vi "Demo_Grab2.vi"() -> ()   [LabVIEW 2024]
doc: "Concurrently grab 2 video sources supported by QuickTime (internal, USB, FW, etc).\nSet Dialogs to 1 in Frame grabber settings to use the standard QT dialog.\n\nChris Salzmann © 1994-2003"
uses:
  <userlib>/ImageProcessing/QTLIB_2595_LV86/QT_Private.ctl
  <userlib>/ImageProcessing/QTLIB_2595_LV86/QT_Video.ctl
  <userlib>/ImageProcessing/QTLIB_2595_LV86/QT_FrameGrabber.ctl
panel:
  in  "Case Constant\n(See Context Help)":bool=TRUE
  in  "Hue 2":dbl(slide)=44.642857142857146 scale=0.0..100.0
  in  "Sat 2":dbl(slide)=39.285714285714285 scale=0.0..100.0
  in  "Bright 2":dbl(slide)=53.06122448979592 scale=0.0..100.0
  in  "Contr 2":dbl(slide)=57.142857142857146 scale=0.0..100.0
  in  "Sharp 2":dbl(slide) scale=0.0..100.0
  in  "Black l. 2":dbl(slide)=10.714285714285715 scale=0.0..100.0
  in  "White l. 2":dbl(slide)=80.61224489795919 scale=0.0..100.0
  out "QT Version 2":string="QuickTime v. 630 "
  out "CIN info 2":string="© Chris 94-2002, QT Fat-CIN, rev: 2576, FATQTCin.c, Jul 11 2003, 11:29:33"
  out "Picture 2":picture
  in  "Frame Grabber Settings 2":T1={"Name"="", "Digitizer"=2, "Input"=1, "Width"=320, "Height"=240, "Input format"=enum."NTSC", "Frame rate"=0.0, "Reserved"=0, "Dialogs"=0} {"Frame rate" format="%#1_6g"; "Dialogs" format="%.0b"}
  out "error out":errorcluster
  in  "White l.":dbl(slide)=80.61224489795919 scale=0.0..100.0
  in  "Black l.":dbl(slide)=51.78571428571429 scale=0.0..100.0
  in  "Sharp":dbl(slide)=12.5 scale=0.0..100.0
  in  "Contr":dbl(slide)=57.142857142857146 scale=0.0..100.0
  in  "Bright":dbl(slide)=53.06122448979592 scale=0.0..100.0
  in  "Sat":dbl(slide)=51.02040816326531 scale=0.0..100.0
  in  "Hue":dbl(slide)=50.0 scale=0.0..100.0
  out "Picture":picture
  in  "stop":bool
  in  "Frame Grabber Settings":T1={"Name"="", "Digitizer"=2, "Input"=0, "Width"=320, "Height"=240, "Input format"=enum."PAL", "Frame rate"=0.0, "Reserved"=0, "Dialogs"=0} {"Frame rate" format="%#1_6g"; "Dialogs" format="%.0b"}
  # "Concurrently grab 2 video sources supported by QuickTime(internal, USB, FW, etc)..\nSet Dialogs to 1 in Frame grabber settings to use the standard QT dialog.\n\nChris Salzmann © 1994-2005"
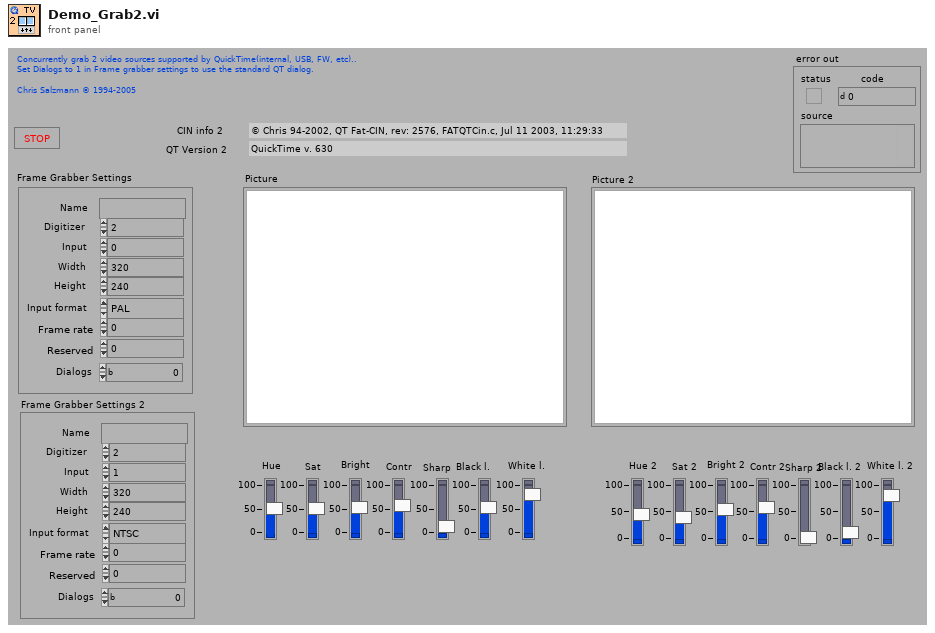
[diagram p1: front panel]
types:
  T1 = typedef "QT_FrameGrabber.ctl" = cluster{"Name":string, "Digitizer":i32, "Input":i32, "Width":i32, "Height":i32, "Input format":enum32{"NTSC", "PAL", "Secam"}, "Frame rate":dbl, "Reserved":i32, "Dialogs":u32}
  T2 = typedef "QT_Video.ctl" = cluster{"Color format":u32, "Hue":dbl, "Saturation":dbl, "Brightness":dbl, "Contrast":dbl, "Sharpness":dbl, "Black Level":dbl, "White Level":dbl, "Options":i32, "Dialogs":u32}
  T3 = typedef "QT_Private.ctl" = cluster{"reserved 1":i32, "reserved 2":i32, "reserved 3":i32, "reserved 4":i32}
  T4 = typedef "QT_Ref.ctl" = refnum<k1>
  T5 = typedef "QT_Image.ctl" = cluster{"Width":i32, "Height":i32, "Depth":i32, "data":u8[], "Compressed data":u8[], "Color table":u32[], "Duration":i32, "Options":i32, "Timestamp":i32, "ID":i32, "Reserved":i32, "Dialogs":u32}
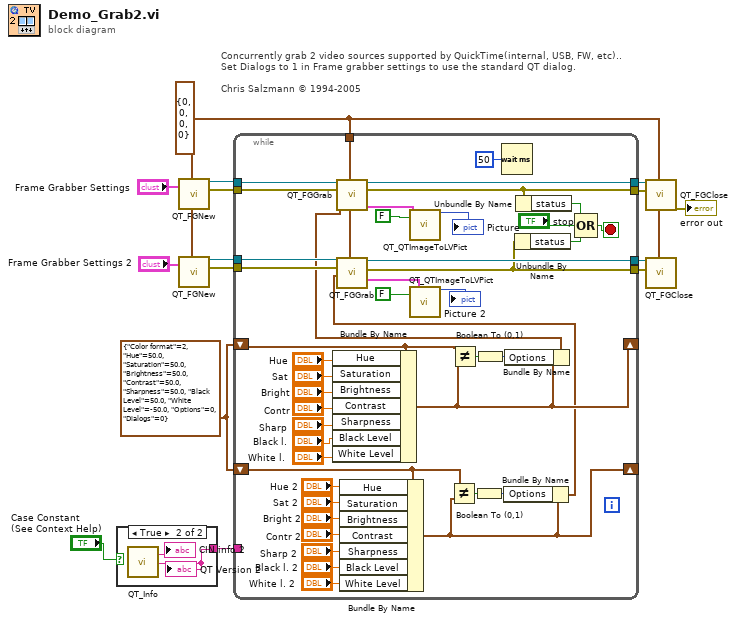
[diagram p0: block diagram]
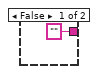
[diagram p2: hidden frame]
diagram:
  w2 = T2 {"Color format"=2, "Hue"=50.0, "Saturation"=50.0, "Brightness"=50.0, "Contrast"=50.0, "Sharpness"=50.0, "Black Level"=50.0, "White Level"=-50.0, "Options"=0, "Dialogs"=0} ("Video Settings")
  w4 = T3 {"reserved 1"=0, "reserved 2"=0, "reserved 3"=0, "reserved 4"=0} ("Private")
  # "Concurrently grab 2 video sources supported by QuickTime(internal, USB, FW, etc)..\nSet Dialogs to 1 in Frame grabber settings to use the standard QT dialog.\n\nChris Salzmann © 1994-2005"
  n1 = case shown="True" "Case Constant\n(See Context Help)" {
    tunnel: ["" ("QT Version") w18] -> w3
    frame False {
    }
    frame True {
      n2 = call <userlib>:"QT_Info.vi"() -> ("CIN info"=→"CIN info 2":string, "QT Version"=w18:string)  [unwired: 3 in, 15 out]
      "QT Version 2" <- w18
    }
  }
  n3 = call <userlib>:"QT_FGNew.vi"("Frame Grabber Settings"="Frame Grabber Settings", "Private"=w4) -> ("QT Ref Out"=w14:T4, "error out"=w12:errorcluster)  [unwired: 3 in, 13 out]
  n4 = call <userlib>:"QT_FGNew.vi"("Frame Grabber Settings"="Frame Grabber Settings 2", "Private"=w4) -> ("QT Ref Out"=w8:T4, "error out"=w5:errorcluster)  [unwired: 3 in, 13 out]
  n5 = while {
    tunnel: w5 -> [w39]
    tunnel: [w32] -> w6
    tunnel: [w40] -> w7
    tunnel: w8 -> [w41]
    shift-left: w2 -> [w45]
    shift-right: [w42] -> _
    tunnel: [w56] -> w11
    tunnel: w12 -> [w59]
    tunnel: w4 -> [w38]
    tunnel: [w61] -> w15
    tunnel: w14 -> [w62]
    tunnel: w3 -> [_]
    shift-right: [w28] -> _
    shift-left: w2 -> [w27]
    stop <- w55 stop-if-true
    n6 = Bundle By Name(cluster=w45, "Hue"="Hue", "Saturation"="Sat", "Brightness"="Bright", "Contrast"="Contr", "Sharpness"="Sharp", "Black Level"="Black l.", "White Level"="White l.") -> (w42:T2)
    n7 = Bundle By Name(cluster=w27, "Hue"="Hue 2", "Saturation"="Sat 2", "Brightness"="Bright 2", "Contrast"="Contr 2", "Sharpness"="Sharp 2", "Black Level"="Black l. 2", "White Level"="White l. 2") -> (w28:T2)
    n8 = Not Equal?(x=w27, y=w28) -> (x != y?=w29:bool)
    n9 = Not Equal?(x=w45, y=w42) -> (x != y?=w44:bool)
    n10 = Boolean To (0,1)(Boolean=w29) -> (0, 1=w30:i16)
    n11 = Boolean To (0,1)(Boolean=w44) -> (0, 1=w43:i16)
    n12 = Wait (ms)(milliseconds to wait=u32 50) -> ()  [unwired: 1 out]
    n13 = Bundle By Name(cluster=w28, "Options"=w30) -> (w26:T2)
    n14 = call <userlib>:"QT_FGGrab.vi"("QT Ref In"=w41, "Video Settings in"=w26, "error in (no error)"=w39, "Private"=w38) -> ("QT Ref Out"=w40:T4, "Image/Movie Out"=w35:T5, "error out"=w32:errorcluster)  [unwired: 2 in, 11 out]
    n15 = call <userlib>:"QT_QTImageToLVPict.vi"("Draw info"=FALSE, "Image/Movie Out"=w35) -> ("Picture color"=→"Picture 2":picture)  [unwired: 1 in, 16 out]
    n16 = Bundle By Name(cluster=w42, "Options"=w43) -> (w37:T2)
    n17 = call <userlib>:"QT_FGGrab.vi"("QT Ref In"=w62, "Video Settings in"=w37, "error in (no error)"=w59, "Private"=w38) -> ("QT Ref Out"=w61:T4, "Image/Movie Out"=w58:T5, "error out"=w56:errorcluster)  [unwired: 2 in, 11 out]
    n18 = call <userlib>:"QT_QTImageToLVPict.vi"("Draw info"=FALSE, "Image/Movie Out"=w58) -> ("Picture color"=→"Picture":picture)  [unwired: 1 in, 16 out]
    n19 = Unbundle By Name(w32) -> ("status"=w31:bool)
    n20 = Unbundle By Name(w56) -> ("status"=w53:bool)
    n21 = Compound Arithmetic op=OR(w53, "stop", w31) -> (w55:bool)
  }
  n22 = call <userlib>:"QT_FGClose.vi"("QT Ref In"=w15, "error in (no error)"=w11, "Private"=w4) -> ("error out"=→"error out":errorcluster)  [unwired: 1 in, 15 out]
  n23 = call <userlib>:"QT_FGClose.vi"("QT Ref In"=w7, "error in (no error)"=w6, "Private"=w4) -> ()  [unwired: 1 in, 16 out]
